vi "Check if boolean value changed.vi"(9 "Var Index":i32, 10 "Values":T1[](array[typedef])) -> (1 "Value":bool, 2 "Value Changed":bool)   [LabVIEW 2011]
uses:
  Measurments Handling/Status Digitalish.ctl
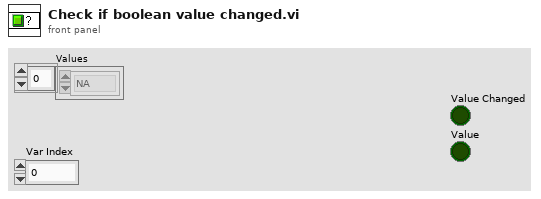
[diagram p1: front panel]
types:
  T1 = typedef "Status Digitalish.ctl" = enum16{"NA", "False", "True"}
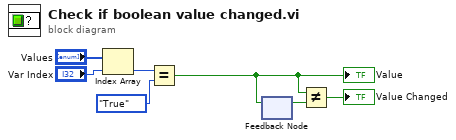
[diagram p0: block diagram]
diagram:
  n1 = Index Array(array="Values", index="Var Index") -> (element=w4:T1)
  n2 = Equal?(x=w4, y=Status_Digitalish."True" ("element")) -> (x = y?=w5:bool)
  "Value" <- w5
  n3 = feedback-in #1(w5) -> ()
  n4 = feedback #1() -> (w7:bool)  [unwired: 1 in]
  n5 = Not Equal?(x=w5, y=w7) -> (x != y?=→"Value Changed":bool)
